vi "DDS update.vi"(8 "error in (no error)":errorcluster, 11 "DDS.lvclass (in)":refnum<class "DDS.lvclass">) -> (0 "error out":errorcluster, 3 "DDS.lvclass":refnum<class "DDS.lvclass">)   [LabVIEW 2014, in "DDS.lvclass"]
uses:
  DDS.lvclass
  DDS.lvclass/DDS.ctl
  Globals.vi
  DDS Library/DDS.lvlib
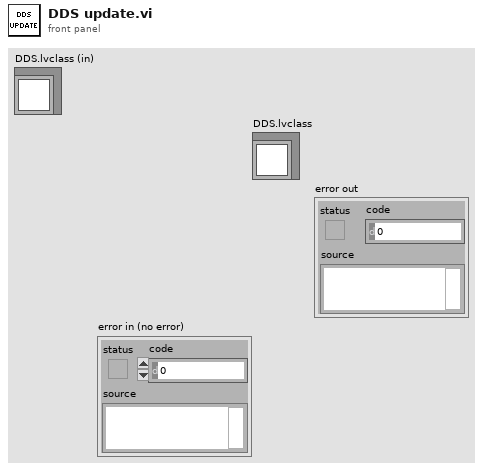
[diagram p1: front panel]
types:
  T1 = typedef "DDS.lvlib/DDS Box Array.ctl" = T2[]
  T2 = typedef "DDS.lvlib/DDS Box Cluster.ctl" = cluster{"DDS box device reference":T3, "Array of DDS Channels (4)":T5, "Enable":bool, "Description":string}
  T3 = typedef "DDS.lvlib/DDS Box Device Reference.ctl" = cluster{"NI USB-8451 device reference":T4, "DIO port":u8, "Serial Clock Rate [kHz]":u16}
  T4 = typedef "ni845xControl.ctl" = refnum<k21>
  T5 = typedef "DDS.lvlib/DDS Channel Array.ctl" = T6[]
  T6 = typedef "DDS.lvlib/DDS Channel.ctl" = cluster{"Power":bool, "Channel Parameters":T7, "RAM Enable":bool, "RAM Dest Type":T8, "RAM Default":cluster{"Frequency [MHz]":dbl, "Amplitude [dBm]":dbl, "Phase Offset [rad]":dbl}, "Array of DDS Profiles (8)":T9, "Description":string}
  T7 = typedef "DDS.lvlib/DDS Channel Parameters.ctl" = cluster{"Ref Clock Rate [MHz]":dbl, "Full Scale Output\nPower [dBm]":dbl}
  T8 = typedef "DDS.lvlib/DDS RAM Destination.ctl" = enum16{"Frequency", "Phase", "Amplitude", "Polar"}
  T9 = typedef "DDS.lvlib/DDS Profile Array.ctl" = T10[]
  T10 = typedef "DDS.lvlib/DDS Profile.ctl" = cluster{"Single Tone":cluster{"Frequency [MHz]":dbl, "Amplitude [dBm]":dbl, "Phase Offset [rad]":dbl}, "RAM Mode ":T11, "Zero-crossing":bool, "No Dwell High":bool, "Function/Static":bool, "RAM Function Settings":string[], "RAM Static Array":dbl[][], "Description":string, "Time Step (us)":T12}
  T11 = typedef "DDS.lvlib/DDS RAM mode.ctl" = enum16{"Direct Switch", "Ramp Up", "Bidirectional Ramp", "Continuous Bidirectional Ramp", "Continuous Recirculate", "Direct Switch 2", "Direct Switch 3", "Direct Switch 4"}
  T12 = typedef "DDS.lvlib/DDS RAM Timestep.ctl" = dbl
  T13 = cluster{"Frequency [MHz]":dbl, "Amplitude [dBm]":dbl, "Phase Offset [rad]":dbl}
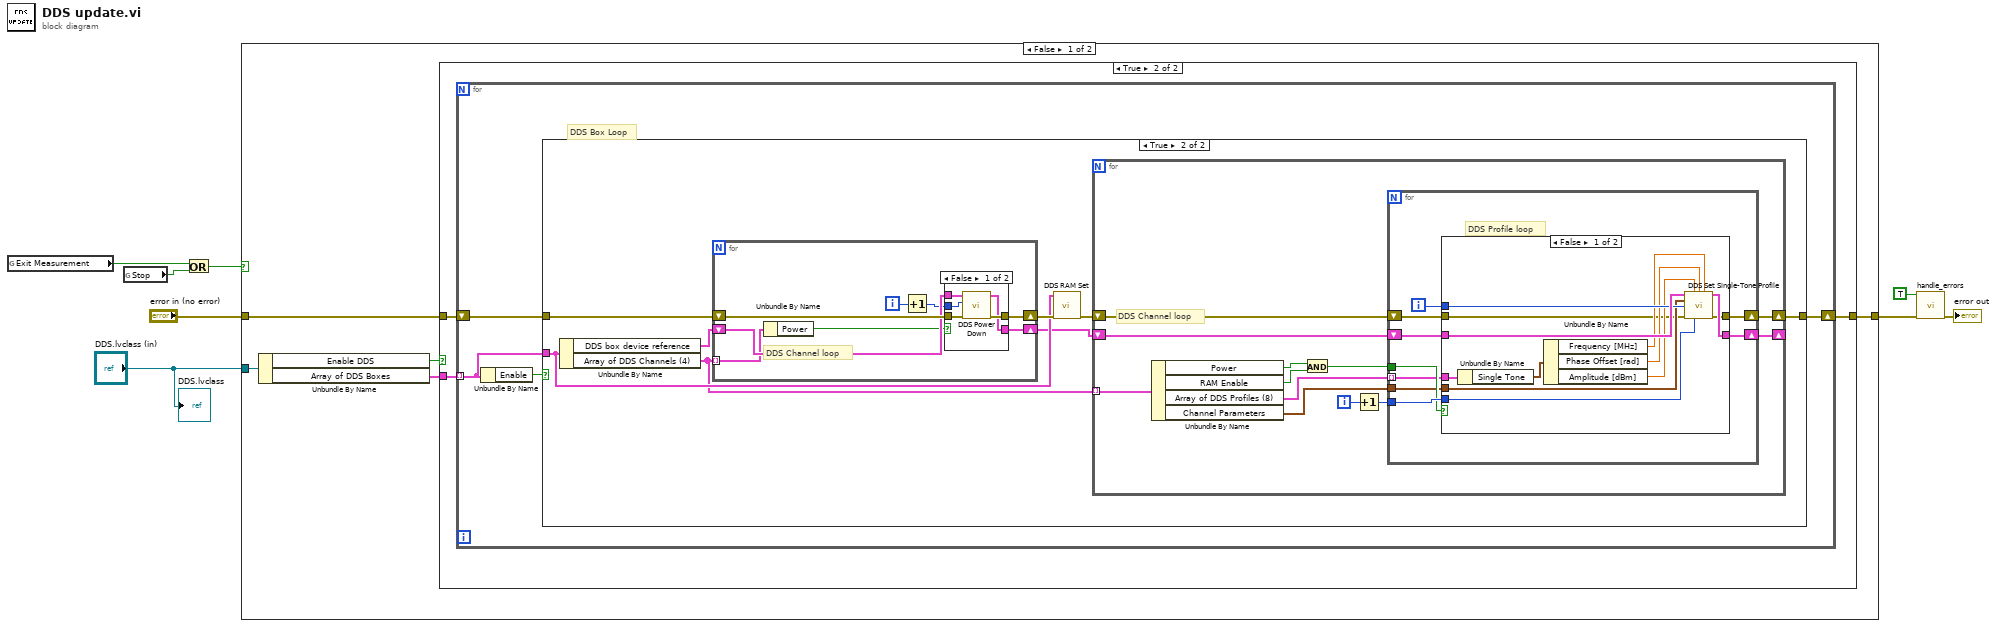
[diagram p0: block diagram]
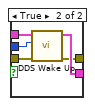
[diagram p5: hidden frame]
diagram:
  n1 = global read "Globals.vi" "Exit Measurement"() -> (w6:bool)
  n2 = global read "Globals.vi" "Stop"() -> (w5:bool)
  n3 = Or(x=w6, y=w5) -> (x .or. y?=w4:bool)
  n4 = case shown="False" w4 {
    tunnel: "error in (no error)" -> [w13 w84]
    tunnel: [w9 w84] -> w2
    tunnel: "DDS.lvclass (in)" -> [w10 _]
    frame False {
      n5 = Unbundle By Name(w10) -> ("Enable DDS"=w12:bool, "Array of DDS Boxes"=w11:T1)
      n6 = case shown="True" w12 {
        tunnel: [w14 w15] -> w9
        tunnel: w13 -> [w14 w17]
        tunnel: w11 -> [_ w16]
        frame False {
        }
        frame True {
          n7 = for {
            shift-right: [w19] -> w15
            shift-left: w17 -> [w18]
            tunnel: w16 -> [w20] mode=indexing
            # "DDS Box Loop"
            n8 = Unbundle By Name(w20) -> ("Enable"=w21:bool)
            n9 = case shown="True" w21 {
              tunnel: w20 -> [_ w27]
              tunnel: w18 -> [w22 w29]
              tunnel: [w22 w24] -> w19
              frame False {
              }
              frame True {
                n10 = Unbundle By Name(w27) -> ("DDS box device reference"=w30:T3, "Array of DDS Channels (4)"=w25:T5)
                n11 = for {
                  shift-right: [w70] -> w23
                  shift-left: w30 -> [w72]
                  shift-right: [w71] -> w28
                  shift-left: w29 -> [w73]
                  tunnel: w25 -> [w67] mode=indexing
                  i -> [w68]
                  # "DDS Channel loop"
                  n12 = Unbundle By Name(w67) -> ("Power"=w66:bool)
                  n13 = Increment(x=w68) -> (x+1=w69:i32)
                  n14 = case shown="False" w66 {
                    tunnel: w73 -> [w78 w83]
                    tunnel: w72 -> [w77 w82]
                    tunnel: [w76 w79] -> w71
                    tunnel: [w75 w80] -> w70
                    tunnel: w69 -> [w74 w81]
                    frame False {
                      n15 = call "DDS Power Down.vi"("error in (no error)"=w78, "chanel number (1)"=w74, "DDS ref in"=w77) -> ("error out"=w76:errorcluster, "DDS ref out"=w75:T3)  [unwired: 7 in]
                    }
                    frame True {
                      n16 = call "DDS Wake Up.vi"("error in (no error)"=w83, "chanel number (1)"=w81, "DDS ref in"=w82) -> ("error out"=w79:errorcluster, "DDS ref out"=w80:T3)  [unwired: 7 in]
                    }
                  }
                }
                n17 = call "DDS RAM Set.vi"("error in (no error)"=w28, "DDS Box Cluster"=w27) -> ("error out"=w26:errorcluster)  [unwired: 8 in, 1 out]
                n18 = for {
                  shift-right: [w41] -> w24
                  shift-left: w26 -> [w31]
                  shift-right: [w40] -> _
                  shift-left: w23 -> [w42]
                  tunnel: w25 -> [w39] mode=indexing
                  i -> [w37]
                  # "DDS Channel loop"
                  n19 = Unbundle By Name(w39) -> ("Power"=w35:bool, "RAM Enable"=w34:bool, "Array of DDS Profiles (8)"=w38:T9, "Channel Parameters"=w32:T7)
                  n20 = And(x=w35, y=w34) -> (x .and. y?=w33:bool)
                  n21 = Increment(x=w37) -> (x+1=w36:i32)
                  n22 = for {
                    shift-right: [w50] -> w40
                    shift-left: w42 -> [w51]
                    shift-right: [w49] -> w41
                    shift-left: w31 -> [w43]
                    tunnel: w33 -> [w46]
                    tunnel: w36 -> [w48]
                    tunnel: w38 -> [w45] mode=indexing
                    tunnel: w32 -> [w44]
                    i -> [w47]
                    # "DDS Profile loop"
                    n23 = case shown="False" w46 {
                      tunnel: w51 -> [w63 w64]
                      tunnel: w43 -> [w52 w65]
                      tunnel: [w62 w64] -> w50
                      tunnel: [w61 w65] -> w49
                      tunnel: w47 -> [w60 _]
                      tunnel: w48 -> [w59 _]
                      tunnel: w45 -> [w58 _]
                      tunnel: w44 -> [w56 _]
                      frame False {
                        n24 = Unbundle By Name(w58) -> ("Single Tone"=w57:T13)
                        n25 = Unbundle By Name(w57) -> ("Frequency [MHz]"=w55:dbl, "Phase Offset [rad]"=w54:dbl, "Amplitude [dBm]"=w53:dbl)
                        n26 = call "DDS Set Single-Tone Profile.vi"("DDS ref in"=w63, "Amplitude [dBm] (0)"=w53, "Phase Offset [rad] (0)"=w54, "Frequency [MHz] (0)"=w55, "Channel Parameters"=w56, "Profile (0)"=w60, "error in (no error)"=w52, "channel number (1)"=w59) -> ("DDS ref out"=w62:T3, "error out"=w61:errorcluster)  [unwired: 5 in, 1 out]
                      }
                      frame True {
                      }
                    }
                  }
                }
              }
            }
          }
        }
      }
    }
    frame True {
    }
  }
  n27 = call "handle_errors.vi"("Exit Operation"=TRUE ("Exit Measurement"), "error in (no error)"=w2) -> ("error out"=→"error out":errorcluster)  [unwired: 13 in]
  "DDS.lvclass" <- "DDS.lvclass (in)"
